vi "FGV_Vision.vi"(6 "Operation":enum16{"Read", "Write"}(ring)=enum."Write", 9 "InVision":T3 {"AntDistance [mm]" format="%_6g"}) -> (3 "OutVision":T3 {"AntDistance [mm]" format="%_6g"})   [LabVIEW 2024]
uses:
  vision/#AntennaControlNumber.ctl
  <vilib>/userDefined/High Color/IMAQdx.ctl
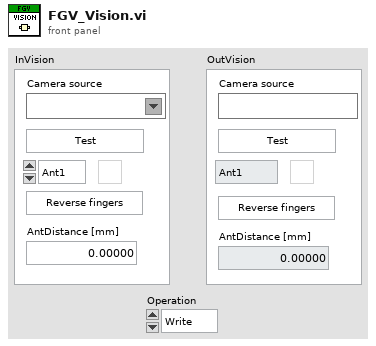
[diagram p1: front panel]
types:
  T1 = typedef "#AntennaControlNumber.ctl" = enum16{"Ant1", "Ant2", "Ant3", "Ant4"}
  T2 = typedef "IMAQdx.ctl" = refnum<k21>
  T3 = cluster{"Reverse fingers":bool, "SelectingButton":bool, "Antenna":T1, "TestVsion":bool, "Camera source":T2, "AntDistance [mm]":dbl}
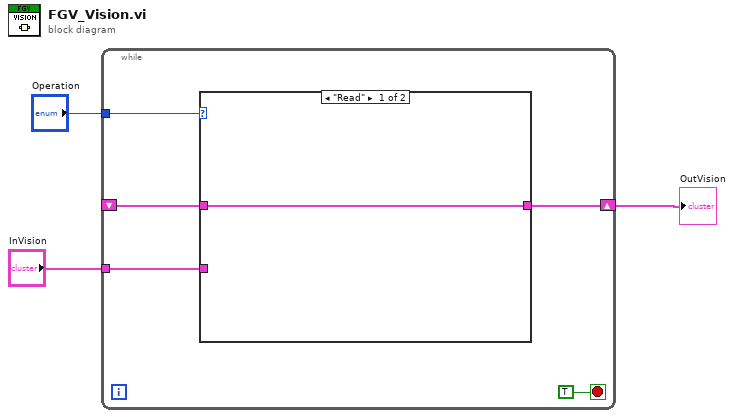
[diagram p0: block diagram]
diagram:
  n1 = while {
    tunnel: "InVision" -> [w8]
    shift-right: [w7] -> w1
    shift-left: _ -> [w6]
    tunnel: "Operation" -> [w5]
    stop <- TRUE stop-if-true
    n2 = case shown="\"Read\"" w5 {
      tunnel: w8 -> [_ w10]
      tunnel: [w9 w10] -> w7
      tunnel: w6 -> [w9 _]
      frame "Read" {
      }
      frame "Write" {
      }
    }
  }
  "OutVision" <- w1
